vi "WriteReductionInfo.vi"(4 "error in (no error)":errorcluster, 5 "# of Entries (before)":i16, 6 "Reduction Info.":T1={"DISPAXIS"=1, "DETSIZE"="[1:4096,1:4096]", "CCDSUM"="1 1", "DETSEC"="[1:4096,1:4096]", "DATASEC"="[1:4096,1:4096]"}, 7 "Path to FITS Header File":path) -> (0 "error out":errorcluster, 2 "# of Entries (after)":i16, 3 "Path to FITS Header File":path)   [LabVIEW 2015]
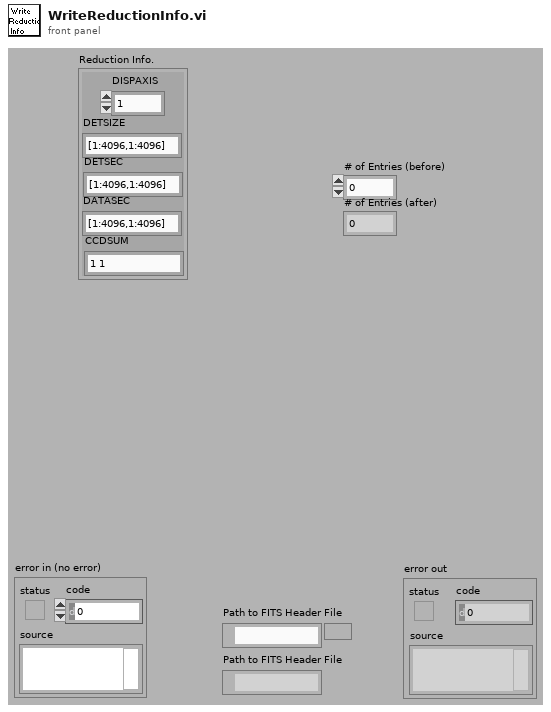
[diagram p1: front panel]
types:
  T1 = cluster{"DISPAXIS":i8, "DETSIZE":string, "CCDSUM":string, "DETSEC":string, "DATASEC":string}
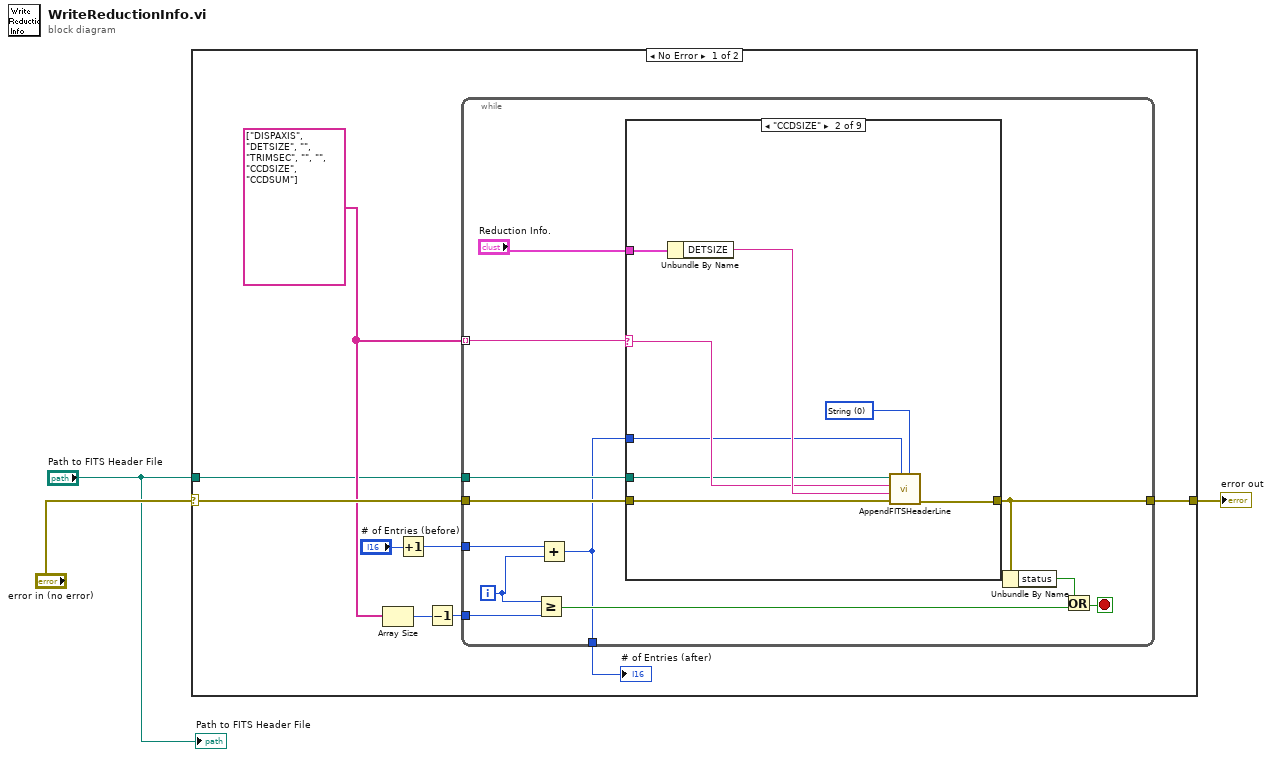
[diagram p0: block diagram]
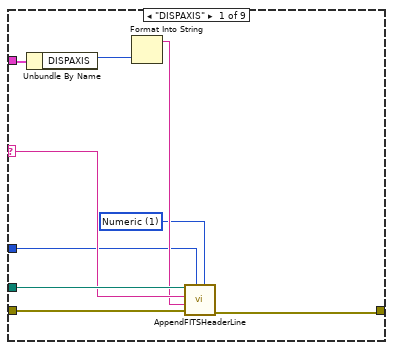
[diagram p2: hidden frame]
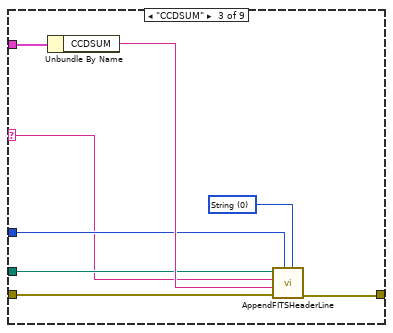
[diagram p3: hidden frame]
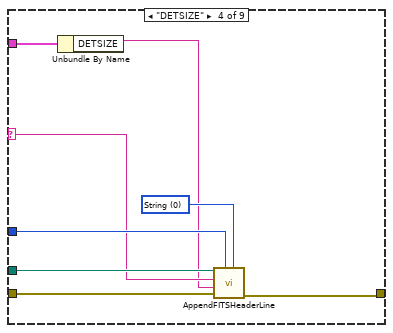
[diagram p4: hidden frame]
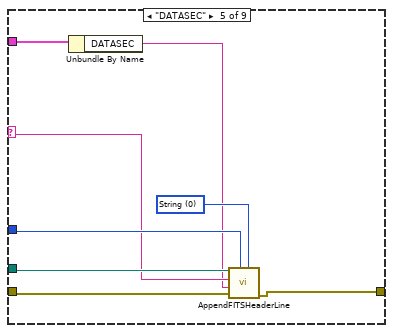
[diagram p5: hidden frame]
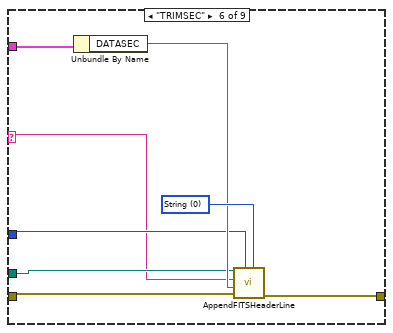
[diagram p6: hidden frame]
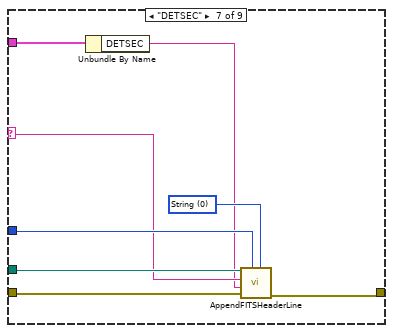
[diagram p7: hidden frame]
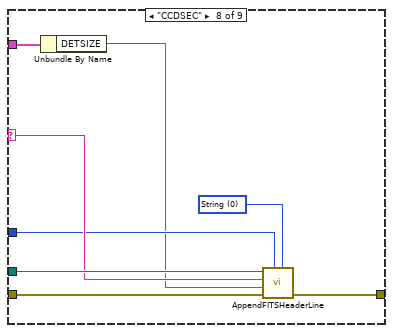
[diagram p8: hidden frame]
diagram:
  n1 = case shown="No Error" "error in (no error)" {
    selector: "error in (no error)" -> [w12 w91]
    tunnel: [w8 w91] -> w2
    tunnel: "Path to FITS Header File" -> [w7 _]
    frame No Error {
      w11 = string[] ["DISPAXIS", "DETSIZE", "", "TRIMSEC", "", "", "CCDSIZE", "CCDSUM"]
      n2 = Array Size(array=w11) -> (size(s)=w10:i32)
      n3 = Increment(x="# of Entries (before)") -> (x+1=w5:i16)
      n4 = Decrement(x=w10) -> (x-1=w9:i32)
      n5 = while {
        tunnel: w12 -> [w24]
        tunnel: w11 -> [w22] mode=indexing
        tunnel: w9 -> [w21]
        tunnel: [w20] -> w8
        tunnel: w7 -> [w17]
        tunnel: w5 -> [w15]
        tunnel: [w14] -> w4
        i -> [w16]
        stop <- w23 stop-if-true
        n6 = Greater Or Equal?(x=w16, y=w21) -> (x >= y?=w19:bool)
        n7 = Add(x=w15, y=w16) -> (x+y=w14:i32)
        n8 = case shown="\"CCDSIZE\"" w22 {
          selector: w22 -> [w30 w38 w44 w52 w61 w68 w77 w85 _]
          tunnel: w24 -> [w33 w35 w47 w53 w64 w71 w80 w88 w90]
          tunnel: [w32 w34 w43 w51 w58 w66 w75 w87 w90] -> w20
          tunnel: "Reduction Info." -> [w26 w39 w42 w56 w59 w67 w76 w89 _]
          tunnel: w17 -> [w31 w36 w46 w54 w63 w70 w79 w86 _]
          tunnel: w14 -> [w27 w37 w45 w55 w62 w69 w78 w83 _]
          frame "DISPAXIS" {
            w28 = u16 1 items=["String", "Numeric", "Boolean"] ("Entry Type")
            n9 = Unbundle By Name(w26) -> ("DISPAXIS"=w25:i8)
            n10 = Format Into String(w25) -> (resulting string=w29:string)  [unwired: 3 in, 1 out]
            n11 = call "AppendFITSHeaderLine.vi"("Entry Type"=w28, "Entry #"=w27, "error in (no error)"=w33, "Element Value"=w29, "Element Name"=w30, "file path (dialog if empty)"=w31) -> ("error out"=w32:errorcluster)  [unwired: 4 in]
          }
          frame "CCDSIZE" {
            w41 = u16 0 items=["String", "Numeric", "Boolean"] ("Entry Type")
            n12 = Unbundle By Name(w39) -> ("DETSIZE"=w40:string)
            n13 = call "AppendFITSHeaderLine.vi"("Entry Type"=w41, "Entry #"=w37, "error in (no error)"=w35, "Element Value"=w40, "Element Name"=w38, "file path (dialog if empty)"=w36) -> ("error out"=w34:errorcluster)  [unwired: 4 in]
          }
          frame "CCDSUM" {
            w49 = u16 0 items=["String", "Numeric", "Boolean"] ("Entry Type")
            n14 = Unbundle By Name(w42) -> ("CCDSUM"=w48:string)
            n15 = call "AppendFITSHeaderLine.vi"("Entry Type"=w49, "Entry #"=w45, "error in (no error)"=w47, "Element Value"=w48, "Element Name"=w44, "file path (dialog if empty)"=w46) -> ("error out"=w43:errorcluster)  [unwired: 4 in]
          }
          frame "DETSIZE" {
            w57 = u16 0 items=["String", "Numeric", "Boolean"] ("Entry Type")
            n16 = Unbundle By Name(w56) -> ("DETSIZE"=w50:string)
            n17 = call "AppendFITSHeaderLine.vi"("Entry Type"=w57, "Entry #"=w55, "error in (no error)"=w53, "Element Value"=w50, "Element Name"=w52, "file path (dialog if empty)"=w54) -> ("error out"=w51:errorcluster)  [unwired: 4 in]
          }
          frame "DATASEC" {
            w65 = u16 0 items=["String", "Numeric", "Boolean"] ("Entry Type")
            n18 = Unbundle By Name(w59) -> ("DATASEC"=w60:string)
            n19 = call "AppendFITSHeaderLine.vi"("Entry Type"=w65, "Entry #"=w62, "error in (no error)"=w64, "Element Value"=w60, "Element Name"=w61, "file path (dialog if empty)"=w63) -> ("error out"=w58:errorcluster)  [unwired: 4 in]
          }
          frame "TRIMSEC" {
            w73 = u16 0 items=["String", "Numeric", "Boolean"] ("Entry Type")
            n20 = Unbundle By Name(w67) -> ("DATASEC"=w72:string)
            n21 = call "AppendFITSHeaderLine.vi"("Entry Type"=w73, "Entry #"=w69, "error in (no error)"=w71, "Element Value"=w72, "Element Name"=w68, "file path (dialog if empty)"=w70) -> ("error out"=w66:errorcluster)  [unwired: 4 in]
          }
          frame "DETSEC" {
            w81 = u16 0 items=["String", "Numeric", "Boolean"] ("Entry Type")
            n22 = Unbundle By Name(w76) -> ("DETSEC"=w74:string)
            n23 = call "AppendFITSHeaderLine.vi"("Entry Type"=w81, "Entry #"=w78, "error in (no error)"=w80, "Element Value"=w74, "Element Name"=w77, "file path (dialog if empty)"=w79) -> ("error out"=w75:errorcluster)  [unwired: 4 in]
          }
          frame "CCDSEC" {
            w84 = u16 0 items=["String", "Numeric", "Boolean"] ("Entry Type")
            n24 = Unbundle By Name(w89) -> ("DETSIZE"=w82:string)
            n25 = call "AppendFITSHeaderLine.vi"("Entry Type"=w84, "Entry #"=w83, "error in (no error)"=w88, "Element Value"=w82, "Element Name"=w85, "file path (dialog if empty)"=w86) -> ("error out"=w87:errorcluster)  [unwired: 4 in]
          }
          frame "", Default {
          }
        }
        n26 = Unbundle By Name(w20) -> ("status"=w18:bool)
        n27 = Or(x=w18, y=w19) -> (x .or. y?=w23:bool)
      }
      "# of Entries (after)" <- w4
    }
    frame Error {
    }
  }
  "error out" <- w2
  "Path to FITS Header File" <- "Path to FITS Header File"
